vi "Write WiFi Config.vi"() -> (0 "error out":errorcluster)   [LabVIEW 2020]
panel:
  in  "Values (other)":dbl[](array[numeric])=[1.0] format="%.2f"
  in  "Names (other)":string[](array[string])=["WIFI_DHCP_ENABLE_DEFAULT"]
  in  "Password":string
  in  "SSID":string="LJOpen"
  in  "IP String Values":string[](array[string])=["192.168.1.217", "255.255.255.0", "192.168.1.1"]
  out "Error String":string
  out "ConnectionType Out":i32
  out "DeviceType Out":i32
  in  "Identifier":string="LJM_idANY"
  in  "ConnectionType":string="LJM_ctANY"
  in  "DeviceType":string="LJM_dtANY"
  out "Values":dbl[](array[numeric]) format="%.2f"
  in  "Names (IP)":string[](array[string])=["WIFI_IP_DEFAULT", "WIFI_SUBNET_DEFAULT", "WIFI_GATEWAY_DEFAULT"]
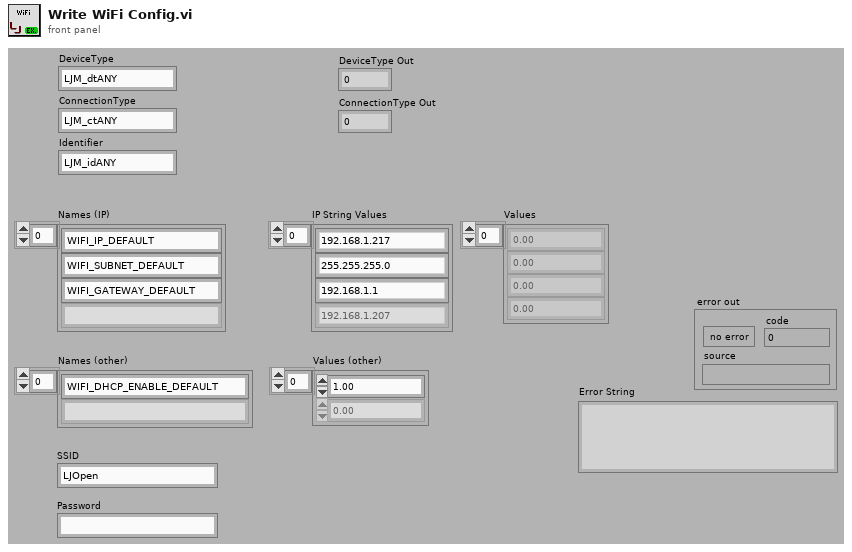
[diagram p1: front panel]
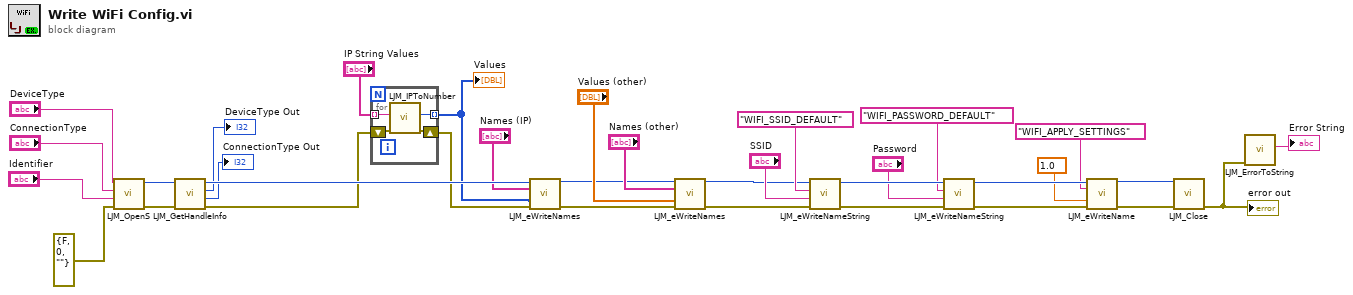
[diagram p0: block diagram]
diagram:
  n1 = call "LJM_OpenS.vi"("error in"=errorcluster {"status"=FALSE, "code"=0, "source"=""} ("error in (no error)"), "Identifier"="Identifier", "ConnectionType"="ConnectionType", "DeviceType"="DeviceType") -> ("error out"=w33:errorcluster, "Handle"=w32:i32)  [unwired: 6 in]
  n2 = call "LJM_GetHandleInfo.vi"("error in"=w33, "Handle In"=w32) -> ("error out"=w19:errorcluster, "ConnectionType"=→"ConnectionType Out":i32, "DeviceType"=→"DeviceType Out":i32, "Handle Out"=w31:i32)  [unwired: 2 in, 4 out]
  n3 = for {
    tunnel: "IP String Values" -> [w38] mode=indexing
    shift-right: [w35] -> w18
    shift-left: w19 -> [w36]
    tunnel: [w37] -> w17 mode=indexing
    n4 = call "LJM_IPToNumber.vi"("error in"=w36, "IPv4String"=w38) -> ("error out"=w35:errorcluster, "Number"=w37:u32)  [unwired: 8 in]
  }
  "Values" <- w17
  n5 = call "LJM_eWriteNames.vi"("Handle In"=w31, "aNames"="Names (IP)", "aValuesIn"=w17, "error in"=w18) -> ("Handle Out"=w3:i32, "error out"=w6:errorcluster)  [unwired: 9 in, 1 out]
  n6 = call "LJM_eWriteNames.vi"("Handle In"=w3, "aNames"="Names (other)", "aValuesIn"="Values (other)", "error in"=w6) -> ("Handle Out"=w2:i32, "error out"=w1:errorcluster)  [unwired: 9 in, 1 out]
  n7 = call "LJM_eWriteNameString.vi"("error in"=w1, "String"="SSID", "Name"="WIFI_SSID_DEFAULT", "Handle In"=w2) -> ("error out"=w21:errorcluster, "Handle Out"=w22:i32)  [unwired: 6 in]
  n8 = call "LJM_eWriteNameString.vi"("error in"=w21, "String"="Password", "Name"="WIFI_PASSWORD_DEFAULT", "Handle In"=w22) -> ("error out"=w11:errorcluster, "Handle Out"=w12:i32)  [unwired: 6 in]
  n9 = call "LJM_eWriteName.vi"("Handle In"=w12, "Name"="WIFI_APPLY_SETTINGS", "Value"=1.0, "error in"=w11) -> ("Handle Out"=w9:i32, "error out"=w10:errorcluster)  [unwired: 10 in]
  n10 = call "LJM_Close.vi"("error in"=w10, "Handle"=w9) -> ("error out"=w25:errorcluster)  [unwired: 9 in]
  "error out" <- w25
  n11 = call "LJM_ErrorToString.vi"("error in"=w25) -> ("String"=→"Error String":string)  [unwired: 10 in]
